vi "VI.vi"() -> ()   [LabVIEW 2010]
panel:
  out "YD3":dbl
  out "YD2":dbl
  out "YD1":dbl
  out "YD0":dbl
  in  "Coordenada_Y":dbl min=0.0 max=2.0
  out "Z_Pos_Ok":bool
  out "Y_Pos_Ok":bool
  out "X_Pos_Ok":bool
  out "Z_Home_Ok":bool
  out "Y_Home_Ok":bool
  out "X_Home_Ok":bool
  in  "ATIVAR AS/RS":bool
  in  "Z_CTRG":bool
  in  "Y_CTRG":bool
  in  "X_CTRG":bool
  in  "Z_HOME":bool
  in  "Y_HOME":bool
  in  "X_HOME":bool
  in  "Start":bool
  in  "Confirmação da posição":bool
  out "ZD3":dbl
  out "ZD2":dbl
  out "ZD1":dbl
  out "ZD0":dbl
  out "XD3":dbl
  out "XD2":dbl
  out "XD1":dbl
  out "XD0":dbl
  out "Posição":dbl
  in  "Coordenada_Z":dbl min=0.0 max=10.0
  in  "Coordenada_X":dbl min=0.0 max=6.0
  out "Esteira 4":bool
  out "Esteira 3":bool
  out "Esteira 2":bool
  out "Esteira 1":bool
  in  "Eletroválvula 4":bool
  in  "Eletroválvula 3":bool
  in  "Eletroválvula 2":bool
  in  "Eletroválvula 1":bool
  out "Sensor 4":bool
  out "Sensor 3":bool
  out "Sensor 2":bool
  out "Sensor 1":bool
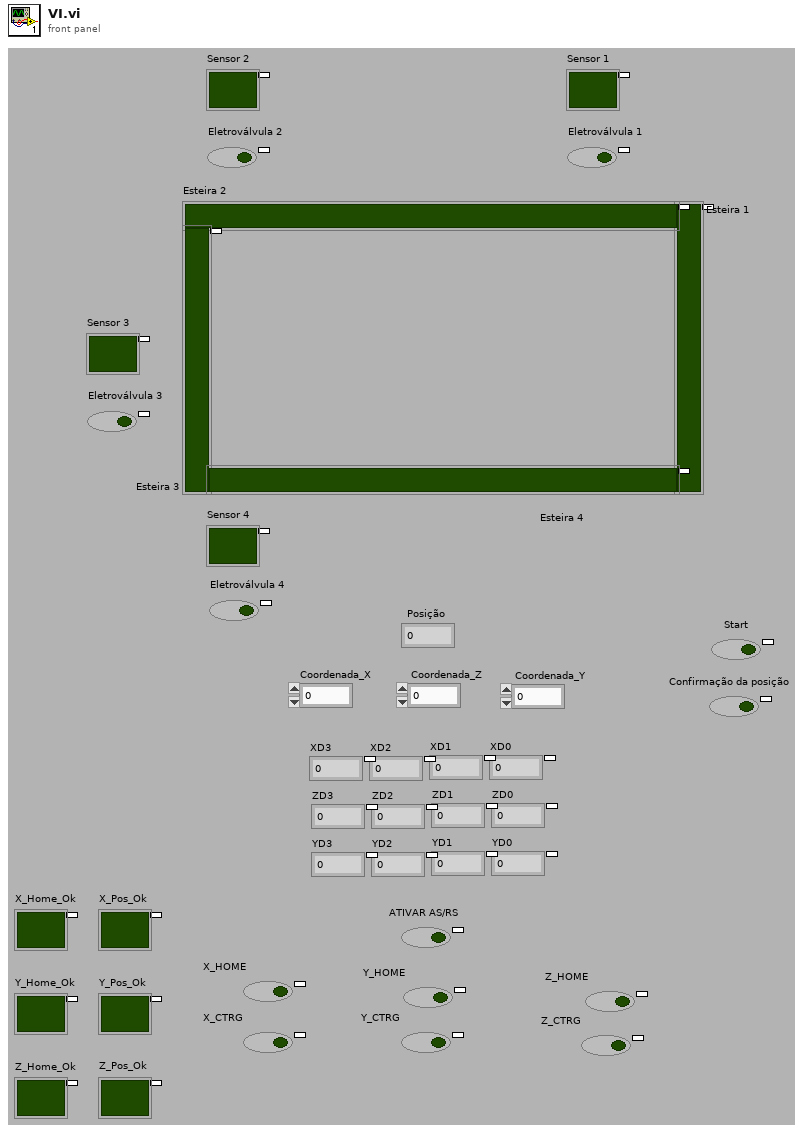
[diagram p1: front panel]
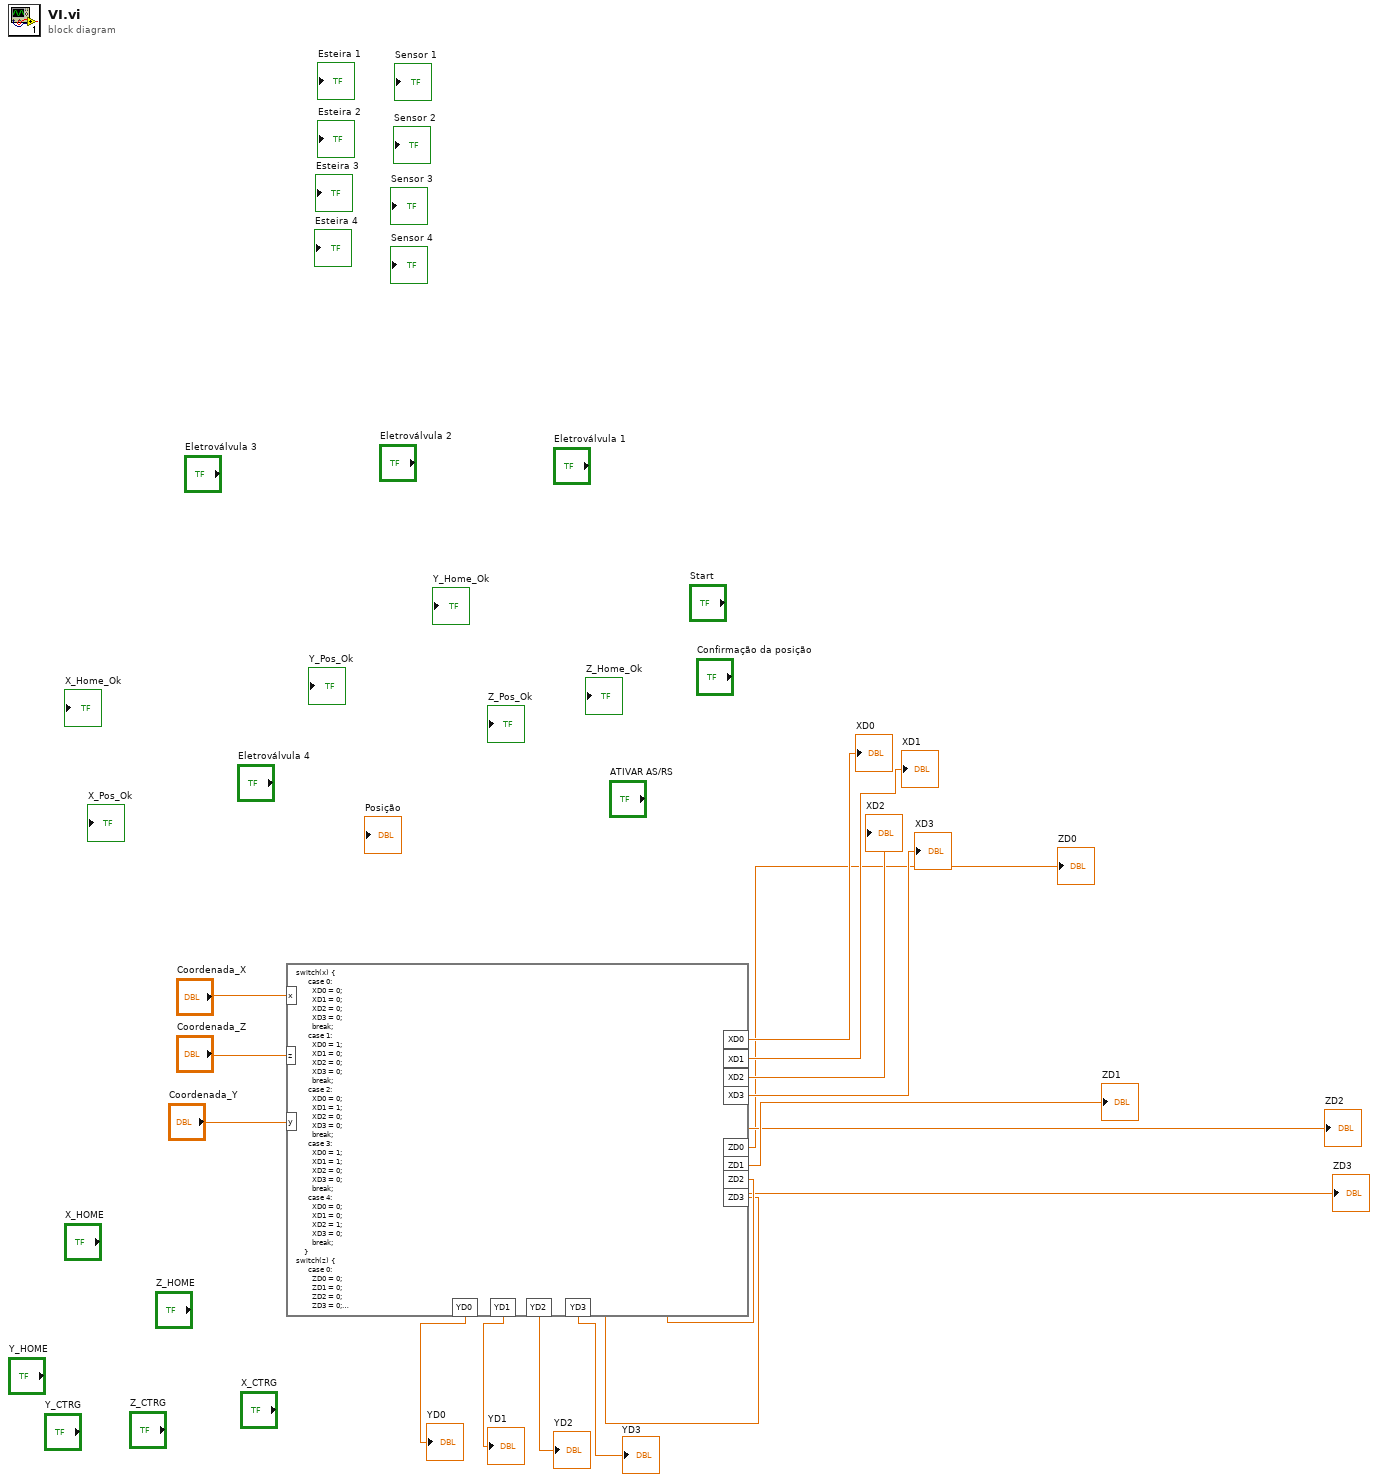
[diagram p0: block diagram]
diagram:
  n1 = formula code="switch(x) {\n      case 0:\n        XD0 = 0;\n        XD1 = 0;\n        XD2 = 0;\n        XD3 = 0;\n        break;\n      case 1: \n        XD0 = 1;\n        XD1 = 0;\n        XD2 = 0;\n        XD3 = 0;\n        break;\n      case 2: \n        XD0 = 0;\n        XD1 = 1;\n        XD2 = 0;\n        XD3 = 0;\n        break;\n      case 3: \n        XD0 = 1;\n        XD1 = 1;\n        XD2 = 0;\n        XD3 = 0;\n        break;\n      case 4: \n        XD0 = 0;\n        XD1 = 0;\n        XD2 = 1;\n        XD3 = 0;\n        break;       \n    }\nswitch(z) {\n      case 0:\n        ZD0 = 0;\n        ZD1 = 0;\n        ZD2 = 0;\n        ZD3 = 0;\n        break;\n      case 1: \n        ZD0 = 1;\n        ZD1 = 0;\n        ZD2 = 0;\n        ZD3 = 0;\n        break;\n      case 2: \n        ZD0 = 0;\n        ZD1 = 1;\n        ZD2 = 0;\n        ZD3 = 0;\n        break;\n      case 3: \n        ZD0 = 1;\n        ZD1 = 1;\n        ZD2 = 0;\n        ZD3 = 0;\n        break;\n      case 4: \n        ZD0 = 0;\n        ZD1 = 0;\n        ZD2 = 1;\n        ZD3 = 0;\n        break; \n      case 5: \n        ZD0 = 1;\n        ZD1 = 0;\n        ZD2 = 1;\n        ZD3 = 0;\n        break; \n      case 6: \n        ZD0 = 0;\n        ZD1 = 1;\n        ZD2 = 1;\n        ZD3 = 0;\n        break; \n      case 7: \n        ZD0 = 1;\n        ZD1 = 1;\n        ZD2 = 1;\n        ZD3 = 0;\n        break; \n      case 8: \n        ZD0 = 0;\n        ZD1 = 0;\n        ZD2 = 0;\n        ZD3 = 1;\n        break; \n      case 9: \n        ZD0 = 1;\n        ZD1 = 0;\n        ZD2 = 0;\n        ZD3 = 1;\n        break; \n      case 10: \n        ZD0 = 0;\n        ZD1 = 1;\n        ZD2 = 0;\n        ZD3 = 1;\n        break; \n      \n    }\n    switch(y) {\n      case 0:\n        YD0 = 0;\n        YD1 = 0;\n        YD2 = 0;\n        YD3 = 0;\n        break;\n      case 1: \n        YD0 = 1;\n        YD1 = 0;\n        YD2 = 0;\n        YD3 = 0;\n        break;\n      case 2: \n        YD0 = 0;\n        YD1 = 1;\n        YD2 = 0;\n        YD3 = 0;\n        break;\n      case 3: \n        YD0 = 1;\n        YD1 = 1;\n        YD2 = 0;\n        YD3 = 0;\n        break;\n      case 4: \n        YD0 = 0;\n        YD1 = 0;\n        YD2 = 1;\n        YD3 = 0;\n        break;       \n    }"("x"="Coordenada_X", "z"="Coordenada_Z", "y"="Coordenada_Y") -> ("XD0"=→"XD0":dbl, "XD1"=→"XD1":dbl, "XD2"=→"XD2":dbl, "XD3"=→"XD3":dbl, "ZD0"=→"ZD0":dbl, "ZD1"=→"ZD1":dbl, "ZD2"=→"ZD2":dbl, "ZD3"=→"ZD3":dbl, "YD0"=→"YD0":dbl, "YD1"=→"YD1":dbl, "YD2"=→"YD2":dbl, "YD3"=→"YD3":dbl)
